vi "Actor.vi"(11 "Actor in":refnum<class "Actor.lvclass">) -> ()   [LabVIEW 2021, in "AAM.lvlib" / "Actor.lvclass"]
uses:
  Actor.lvclass
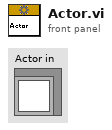
[diagram p1: front panel]
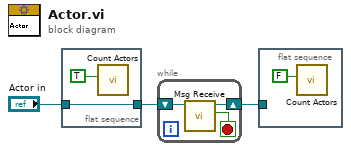
[diagram p0: block diagram]
diagram:
  n1 = flat-sequence {
    tunnel: [w5] -> w3
    tunnel: "Actor in" -> [w5]
    frame #0 {
      n2 = call "Count Actors.vi"("Increment?"=TRUE) -> ()  [unwired: 11 in]
    }
  }
  n3 = while {
    shift-right: [w7] -> w2
    shift-left: w3 -> [w6]
    stop <- w8 stop-if-true
    n4 = call-dynamic "Msg Receive.vi"("Msg Receive in"=w6) -> ("Destroy Self?"=w8:bool, "Actor out"=w7:refnum<class "Actor.lvclass">)  [unwired: 9 in]
  }
  n5 = flat-sequence {
    tunnel: w2 -> [_]
    frame #0 {
      n6 = call "Count Actors.vi"("Increment?"=FALSE) -> ()  [unwired: 11 in]
    }
  }
